vi "store variable by name.vi"(8 "error in":errorcluster, 9 "varient in":variant, 10 "Variable Name":string, 11 "refnum in":T1) -> (0 "error out":errorcluster, 1 "value changed?":bool, 2 "variable already exists?":bool, 3 "refnum out":T1)   [LabVIEW 2020, in "Publisher Subscriber.lvlib"]
uses:
  Publisher Subscriber.lvlib
  Controls/node refnum.ctl
  Controls/node dvr data.ctl
  Controls/data cluster.ctl
  Controls/subscription bank ref.ctl
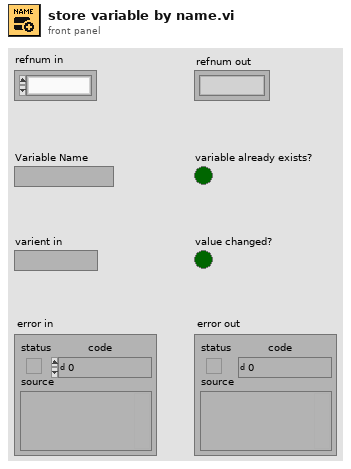
[diagram p1: front panel]
types:
  T1 = typedef "Publisher Subscriber.lvlib/node refnum.ctl" = refnum<k1>
  T2 = typedef "Publisher Subscriber.lvlib/node dvr data.ctl" = cluster{"queue ref":refnum<queue>, "Subscription Bank Ref":refnum<data-value>, "Command":string, "Data":variant, "Subscriptions []":set{string}, "Variables DVR Ref":refnum<data-value>}
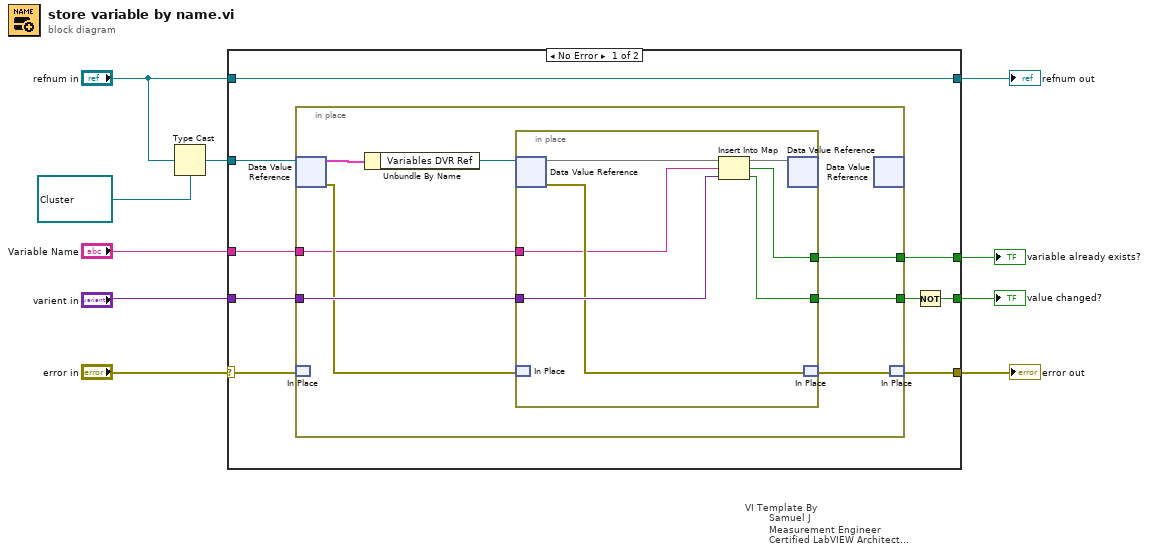
[diagram p0: block diagram]
diagram:
  n1 = Type Cast(type=refnum<data-value> refnum ("data value reference"), x="refnum in") -> (*(type *) &x=w7:refnum<data-value>)
  n2 = case "VI Template By\n        Samuel J\n        Measurement Engineer\n        Certified LabVIEW Architect\n        Vestas Technology R&D Chennai" shown="No Error" "error in" {
    selector: "error in" -> [w17 w36]
    tunnel: [w16 w36] -> w9
    tunnel: w7 -> [w18 _]
    tunnel: [w19 w35] -> w6
    tunnel: "refnum in" -> [w19 w35]
    tunnel: "varient in" -> [w15 _]
    tunnel: "Variable Name" -> [w14 _]
    tunnel: [w13 _] -> w2
    tunnel: [w11 _] -> w1
    frame No Error {
      n3 = in-place {
        in-place-border: w15 -> [w25]
        in-place-border: w14 -> [w22]
        in-place-border: [w21] -> w13
        in-place-border: [w20] -> w12
        n4 = in-place-dvr #1(w18) -> (w27:T2, w24:errorcluster)
        n5 = in-place-match #2(w17) -> ()  [unwired: 1 out]
        n6 = Unbundle By Name(w27) -> ("Variables DVR Ref"=w26:refnum<data-value>)
        n7 = in-place {
          in-place-border: w25 -> [w32]
          in-place-border: w22 -> [w30]
          in-place-border: [w29] -> w21
          in-place-border: [w28] -> w20
          n8 = in-place-dvr #3(w26) -> (w34:map{string, variant}, w31:errorcluster)
          n9 = in-place-match #4(w24) -> ()  [unwired: 1 out]
          n10 = Insert Into Map(map in=w34, key=w30, value=w32) -> (map out=w33:map{string, variant}, key already included?=w29:bool, value unchanged?=w28:bool)
          n11 = in-place-dvr #3(w33) -> ()  [unwired: 2 out]
          n12 = in-place-match #4(w31) -> (w23:errorcluster)
        }
        n13 = in-place-dvr #1() -> ()  [unwired: 1 in, 2 out]
        n14 = in-place-match #2(w23) -> (w16:errorcluster)
      }
      n15 = Not(x=w12) -> (.not. x?=w11:bool)
    }
    frame Error {
    }
  }
  "error out" <- w9
  "refnum out" <- w6
  "variable already exists?" <- w2
  "value changed?" <- w1
